vi "DelayFind.vi"() -> ()   [LabVIEW 2020]
doc: "Example Description:\nThis example demonstrates how to enable Time Interleaved Sampling with the NI 5772 adapter module to achieve a sampling rate of 1.6GS/s. This example continuously acquires records of analog input data from the NI 5772 adapter module. It allows you to select an AI channel, trigger type, and record size. This VI must be compiled before it is run. \n\nVI Configuration:\nThis example uses the NI PXI-7952R as the FPGA target by default. If you are using another FPGA target, complete the following steps to configure the host VI to use a VI configured for your FPGA target:\n1. On the block diagram, right-click the Open FPGA VI Reference (NI PXI-7952R) function and select Configure Open FPGA VI Reference.\n2. Browse for a new target by clicking the Browse Project button in the Open VI section.\n3. Select the VI under the target that matches your device. Click OK to select this VI.\n4. Click OK to exit the dialog box and to apply the new selection to the FPGA VI.\n5. Save the VI.\n\nRunning the VI:\n1. Select a RIO Resource that corresponds to the FPGA device configured above.\n2. Clock Configuration: Select the desired clock source for the adapter module.\nAnalog Input: Configure the AI Channel, Record Size, and Trigger Type controls. If you are using the analog trigger type, configure the Trigger Level (V) control.\n3. Click the run arrow to run the VI.\n4. If the Trigger Type is set to Software, click the Software Trigger button to acquire a single record of data. If the Trigger Type is set to Data Edge, a record of data is acquired each time the input signal rises above the trigger level.\n\nThe Record Size, Trigger Type, and Trigger Level (V) controls can all be configured while the VI is running. \n\nNote: The AI Channel control must be configured before the VI is run.\n\nExecution Steps:s\n1. Open a session to the FPGA VI and run the VI.\n2. Wait for the adapter module to load its default configuration.\n3. Configure the NI 5772 for Time Interleaved Sampling (TIS)\n4. The Trigger type and record size for a single record acquisition are configured.\n5. Based on the trigger type, either wait for the software trigger Boolean to assert or configure the desired trigger level and arm the trigger.\n6. After the trigger is armed, a single record of data is acquired and read.\n7. Stop the VI when the stop button is pressed or when an error has occurred. \n8. Close the FPGA VI reference and display any errors."
uses:
  <vilib>/rvi/interface/nirviCloseFPGA/nirviCloseFPGA.xnode
  SubVIs/DigiFPGARef.ctl
  <vilib>/FPGAPlugInAG/Dynamic/niLvFpga_Close_Dynamic.vi
  Gen/Generator_States.ctl
  <instrlib>/_niInstr/Basic Elements/v1/FPGA/niInstr Basic Elements v1 FPGA.lvlib
  Digitizer_StatesMain.ctl
  <vilib>/rvi/interface/nirviReadWriteControl/nirviReadWriteControl.xnode
  <vilib>/rvi/interface/Simulation/niFpgaSimulationCallBeginRW.vi
  <vilib>/rvi/errors/niLvFpgaAdjustHostInterfaceError.vi
  <vilib>/userdefined/High Color/nirio_resource_hc.ctl
panel:
  out "Trigger Count":u32
  out "Digitizer On":bool
  in  "Amplitude Range":cluster{"Slider 1":dbl, "Slider 1":dbl}(slide)={"Slider 1"=1.0, "Slider 1"=1.6299559471365639} scale=-2.5..2.5
  in  "Range":dbl=2.0
  in  "FineDelay  Control":dbl(slide)=1.0 scale=-2.0..2.0
  in  "Amplitude \nAveraging":u16(slide)=1 caption="Amplitude Averaging" scale=0.0..8.0 scale format="%#.2g"
  in  "Time Division":u8(slide)=1 max=2 step=1 scale=0.0..2.0
  out "Gen Actual Sample Rate":dbl format="%#_6p"
  out "TIS Configured?":bool
  out "Configured?":bool
  in  "Record Size":u16=1024
  in  "Delay(us)":sgl min=0 step=0.1 format="%#_4g"
  in  "TrigIn_Sim":bool caption="Pause"
  out "Waveform LIVE":cluster{"Start Time":dbl, dbl, ext[]}(graph)
  in  "Start Digi":bool
  out "Input Waveform 2":waveform(dbl)(graph)
  out "TimeDivFactor":i16
  out "Read Size (Host)":u16
  out "range (Vpp)":dbl=1.3
  out "FPGA VI Reference Out":T1
  in  "Start Gen":bool
  out "Generator On":bool
  out "Input Waveform":dbl[](graph)
  in  "stop Gen":bool
  in  "Stop Generator \nApplication":bool
  out "Waves per Pixel":u32
  out "Sampling Frequency (Hz)":u64
  out "Amplitudes":dbl[](array[numeric]) format="%.2f"
  out "Offset Factor":dbl
  out "Gain":dbl
  in  "Use Default Wave Settings":bool caption="Checkbox"
  in  "Generator Resource":refnum<k15>
  in  "nGenTrig/vi":bool=TRUE caption="Trigger Mode"
  in  "Digi RIO Resource":T2="PXI1Slot2"
  in  "Ext/nViTrig":bool=TRUE
  in  "Send vi Trig":bool
  in  "Trigger Level (V)":dbl
  out "WaveSampleCount":i16=1024
  out "AvgCount_powerOf2":i16(knob) caption="Amplitude Avg" min=0 max=8 step=1 scale=0.0..8.0
  in  "Stop Digi App":bool caption="Stop Digi \nApplication"
  in  "Trigger Type":enum8{"Software", "Data Edge"}(ring)
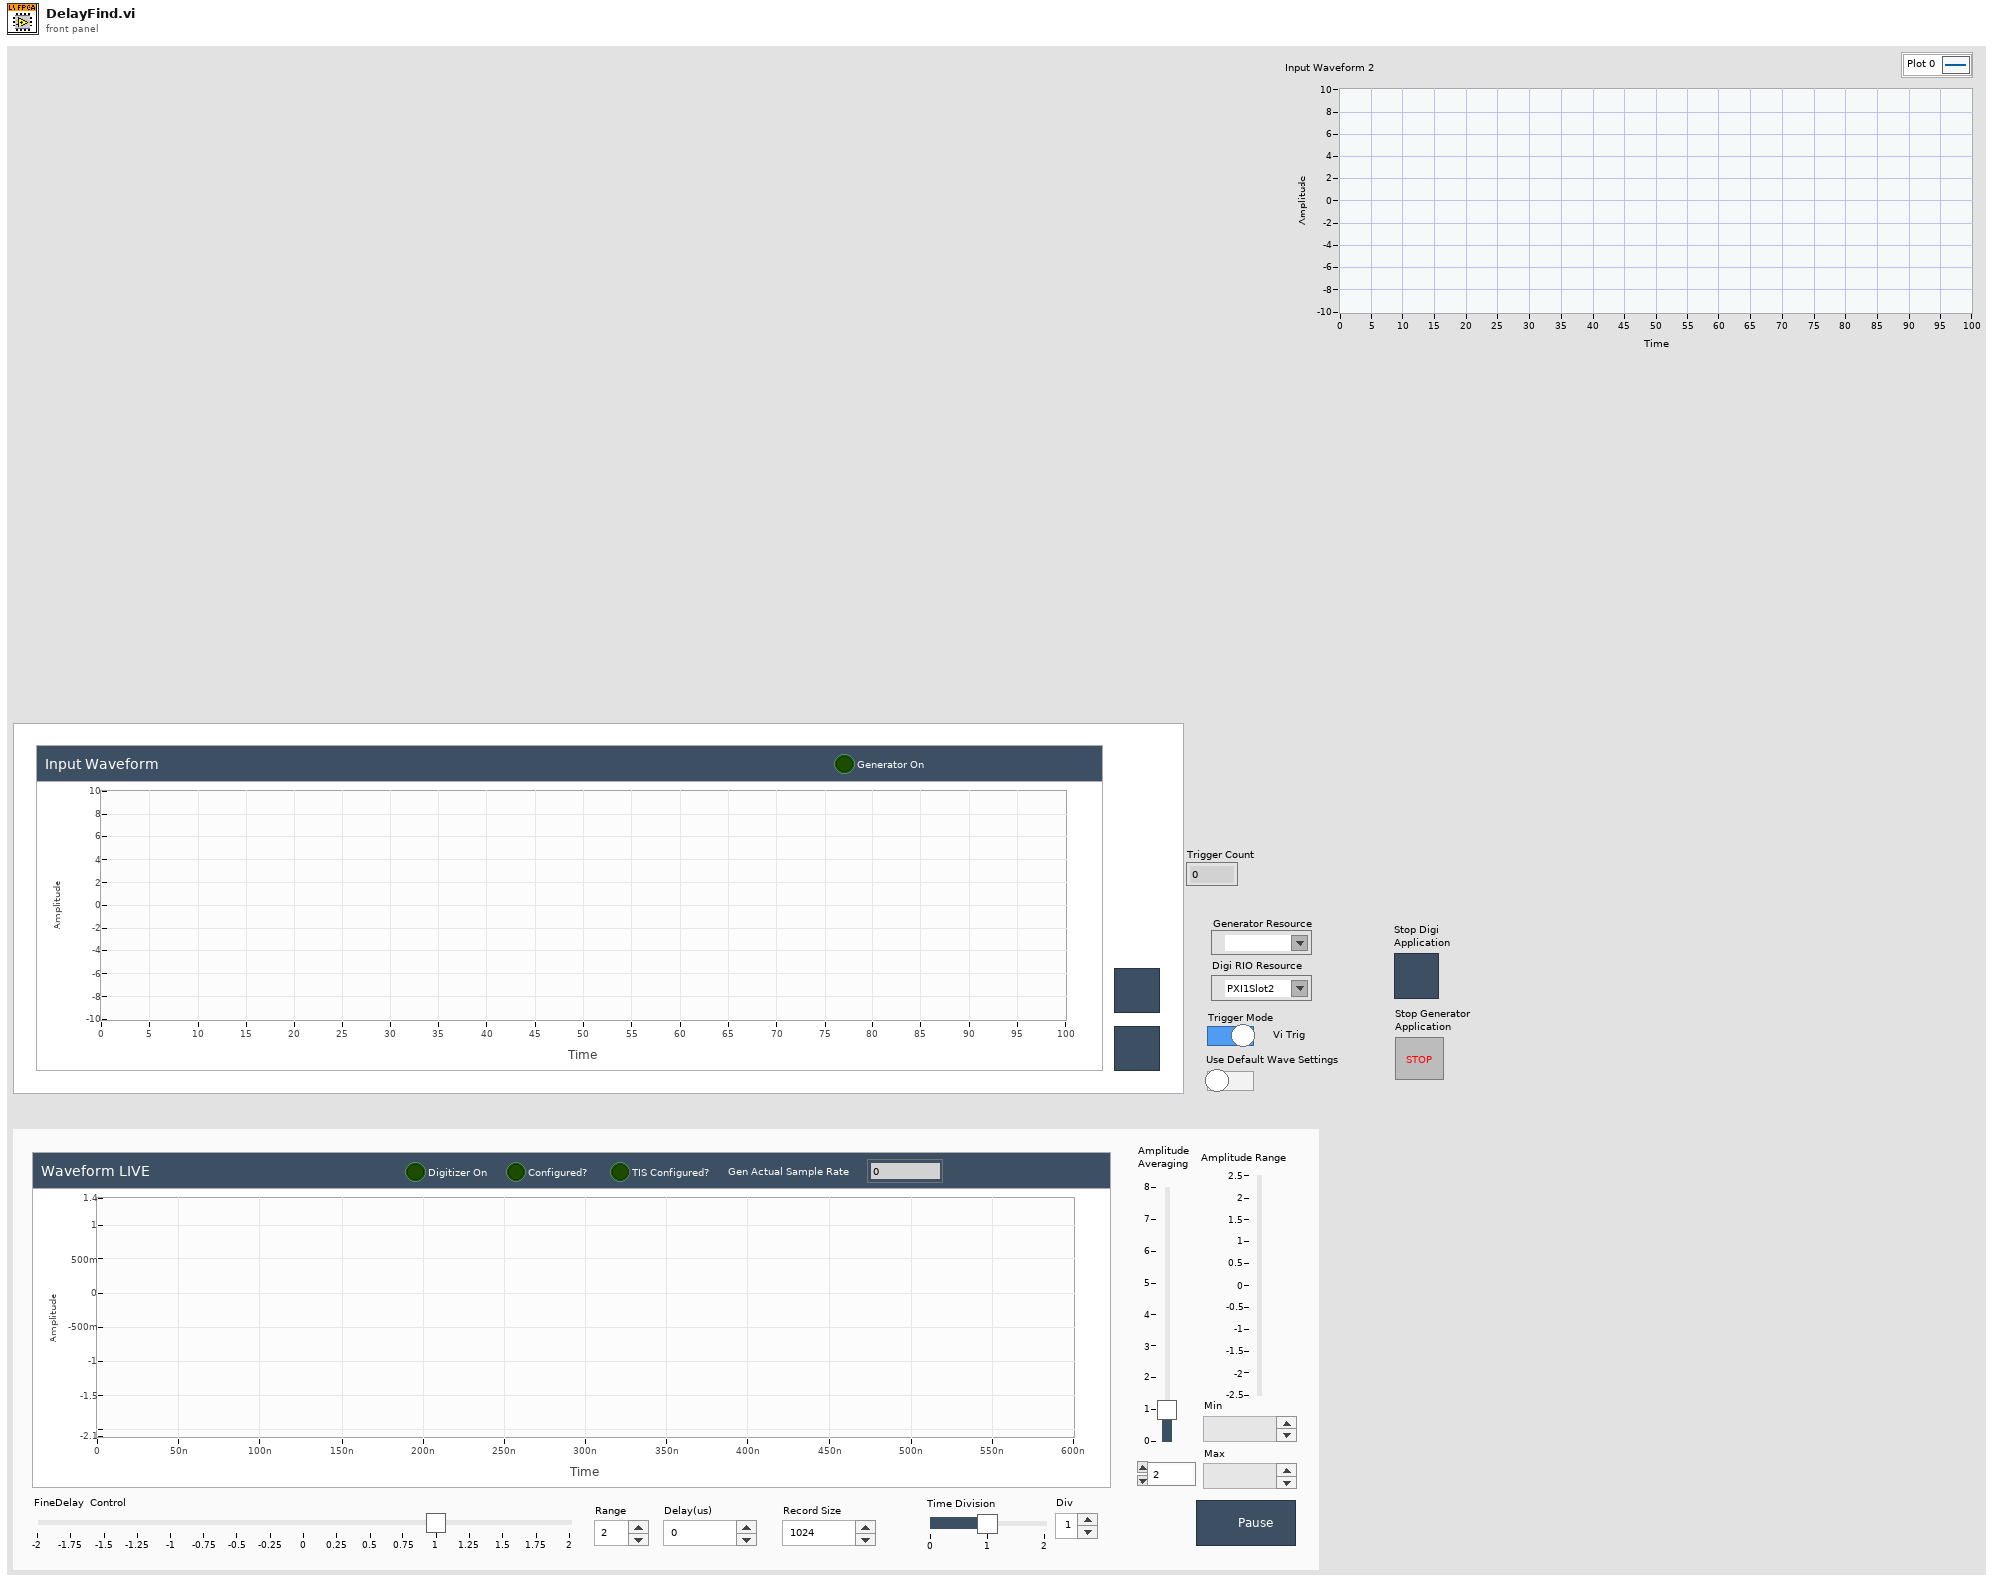
[diagram p1: front panel]
types:
  T1 = typedef "DigiFPGARef.ctl" = refnum<k20>
  T2 = typedef "nirio_resource_hc.ctl" = tag
  T3 = typedef "Digitizer_StatesMain.ctl" = enum16{"Idle", "Init", "SetParam", "Read", "CloseDigi", "CloseApp"}
  T4 = typedef "Generator_States.ctl" = enum16{"Idle", "GenerateWaveArray", "InitGen", "SendVITrig", "CloseGen", "CloseApp"}
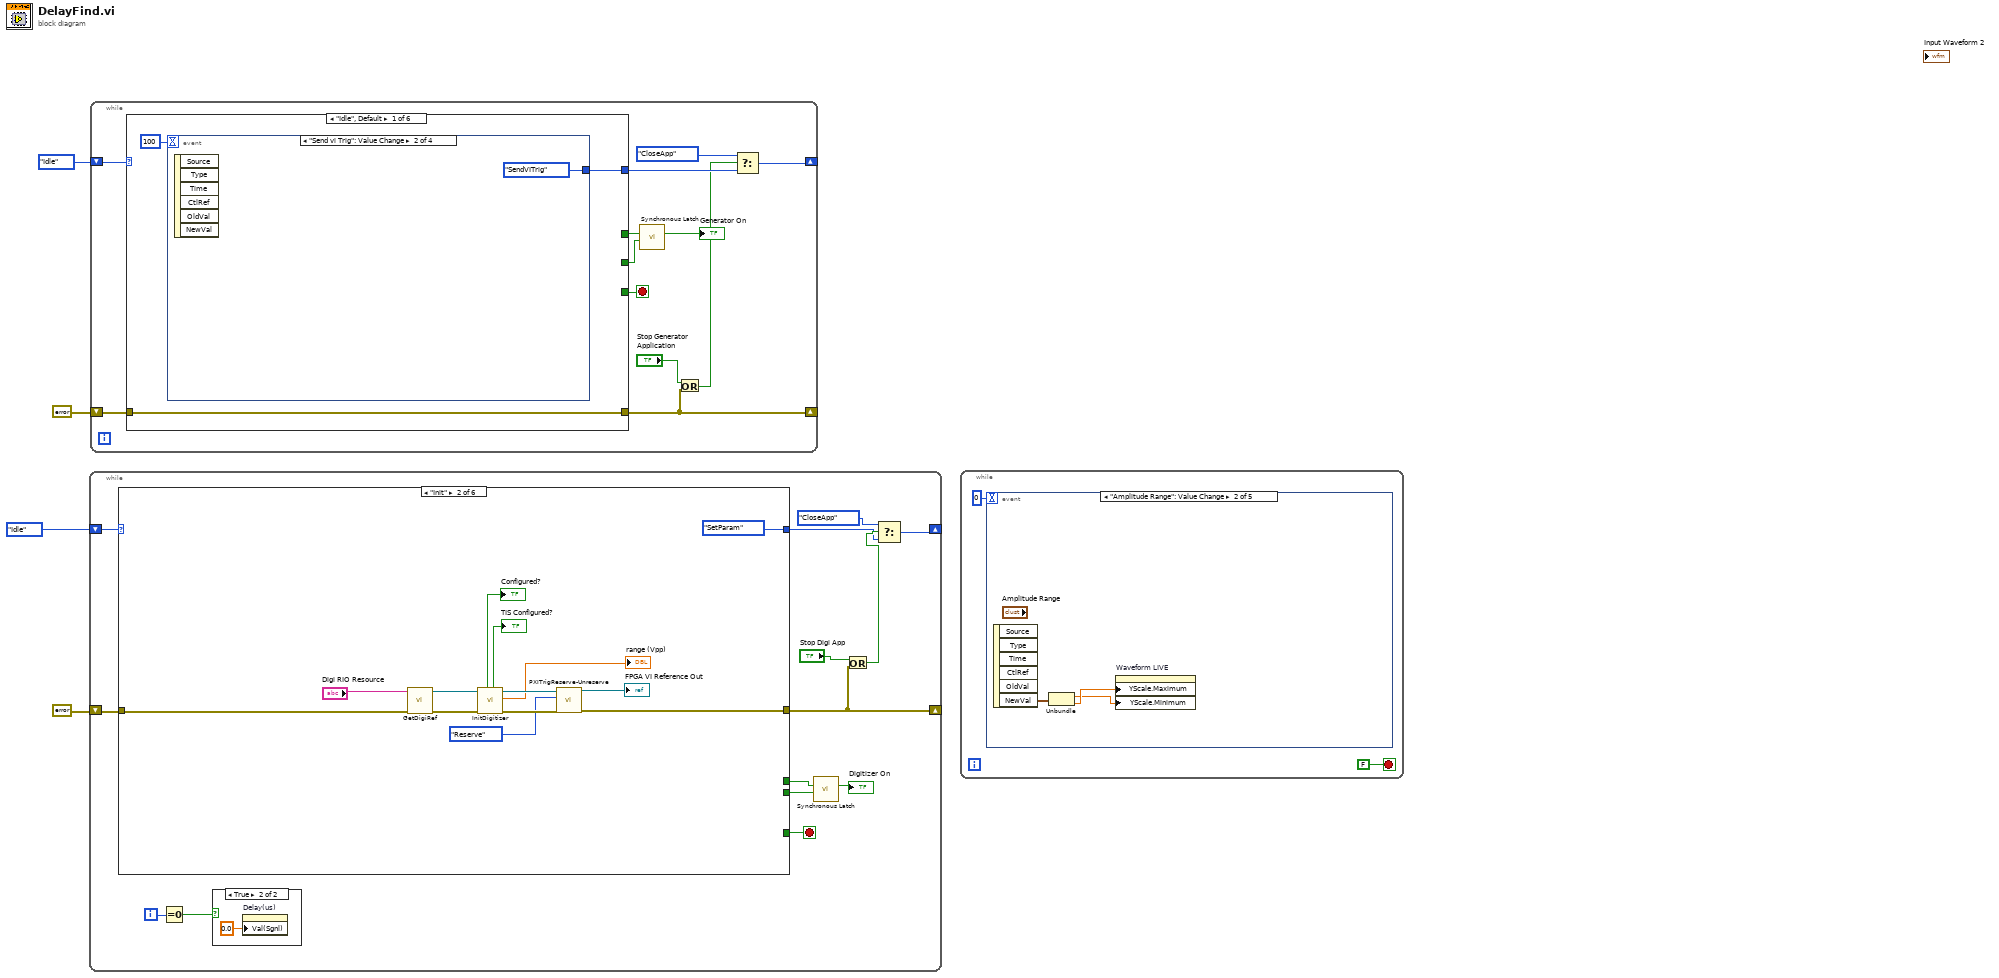
[diagram p0: block diagram]
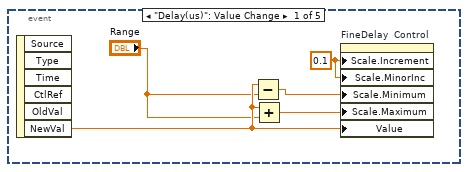
[diagram p2: hidden frame]
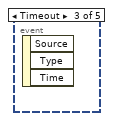
[diagram p3: hidden frame]
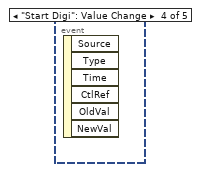
[diagram p4: hidden frame]
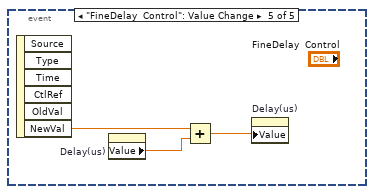
[diagram p5: hidden frame]
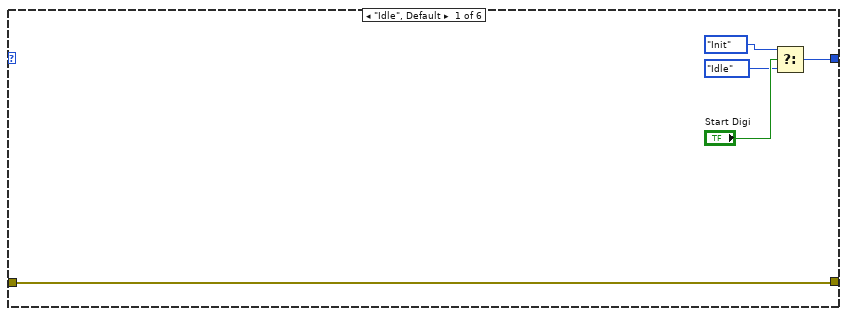
[diagram p7: hidden frame]
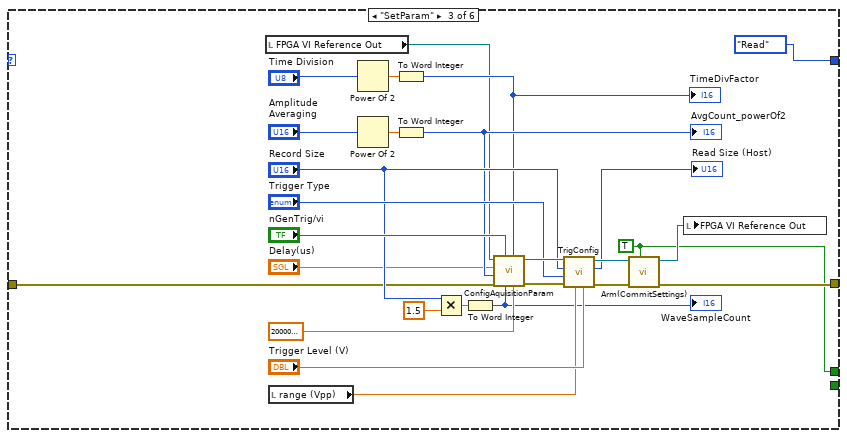
[diagram p8: hidden frame]
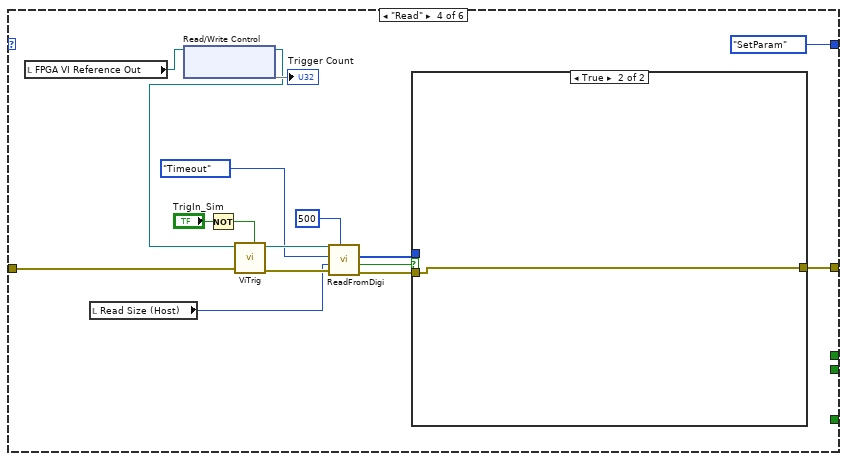
[diagram p9: hidden frame]
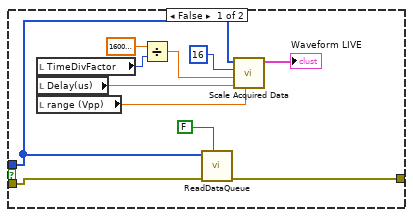
[diagram p10: hidden frame]
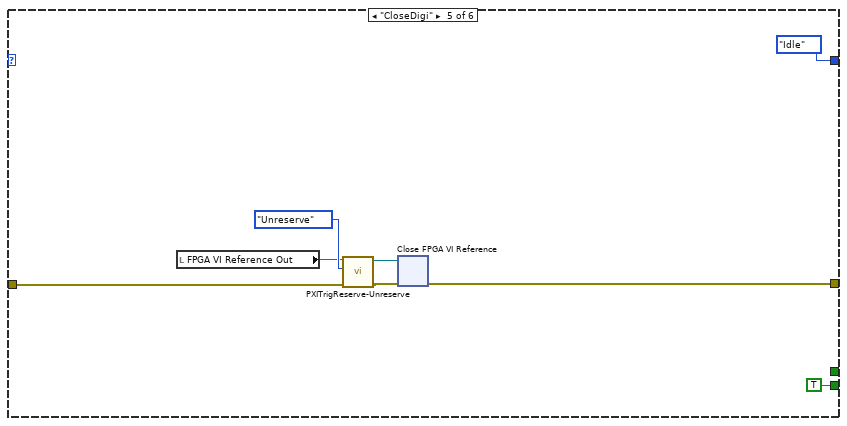
[diagram p11: hidden frame]
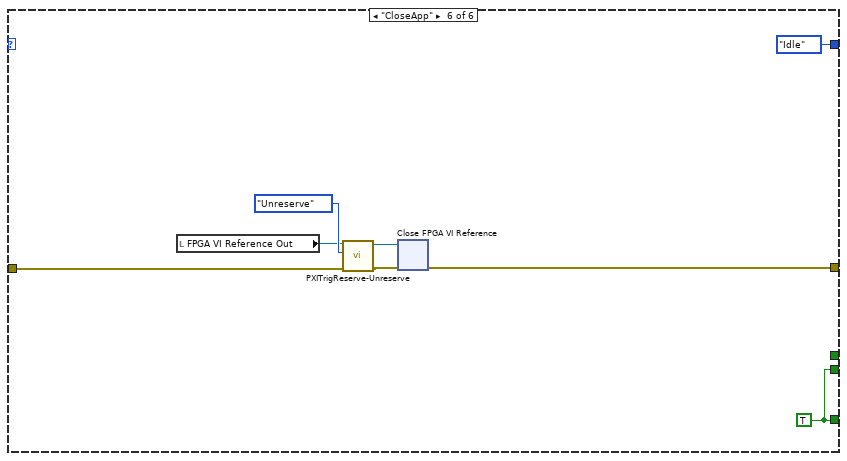
[diagram p12: hidden frame]
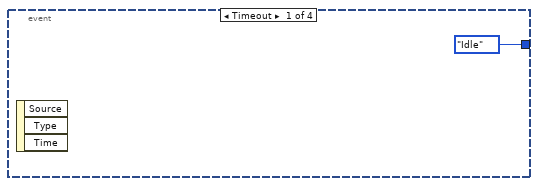
[diagram p13: hidden frame]
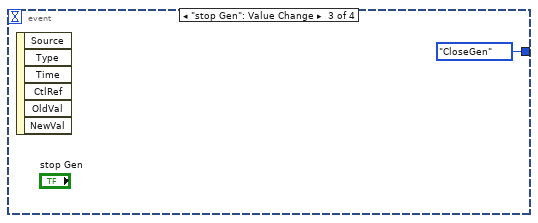
[diagram p14: hidden frame]
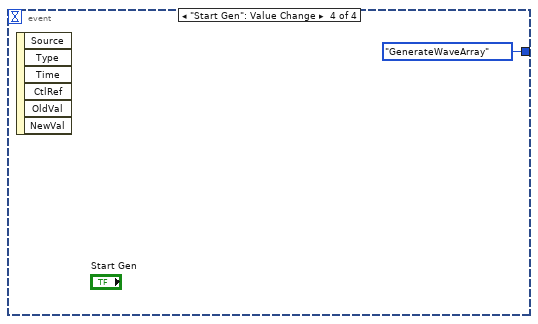
[diagram p15: hidden frame]
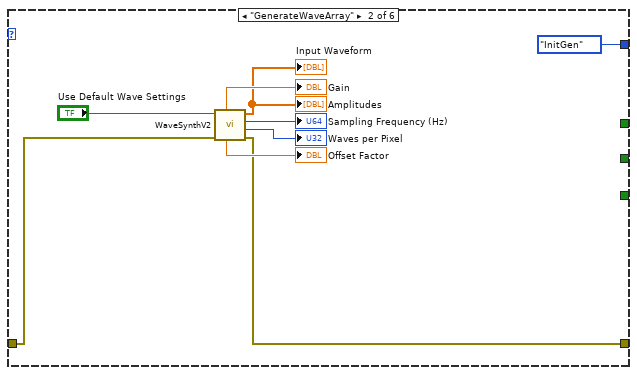
[diagram p16: hidden frame]
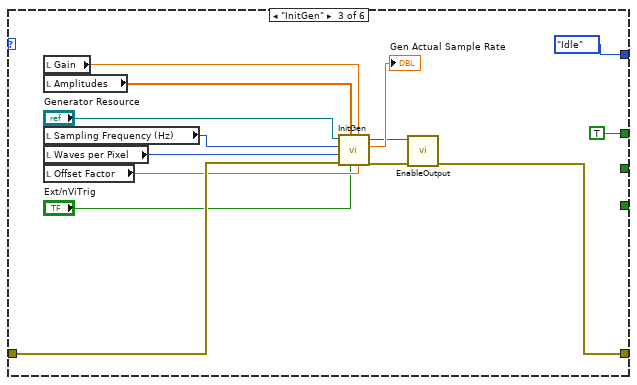
[diagram p17: hidden frame]
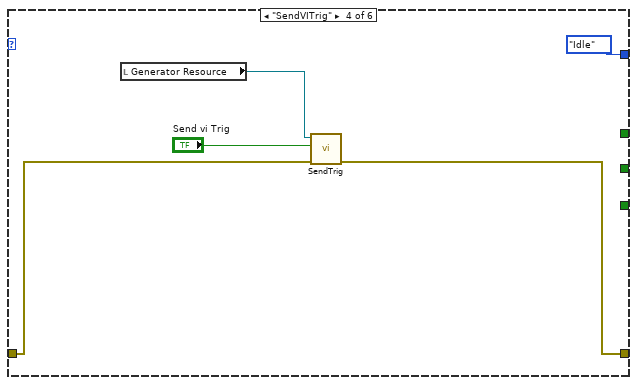
[diagram p18: hidden frame]
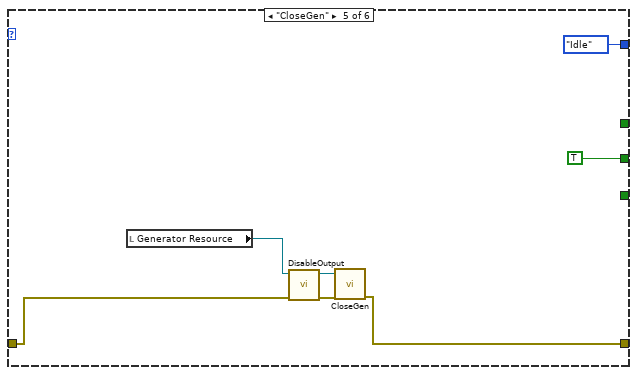
[diagram p19: hidden frame]
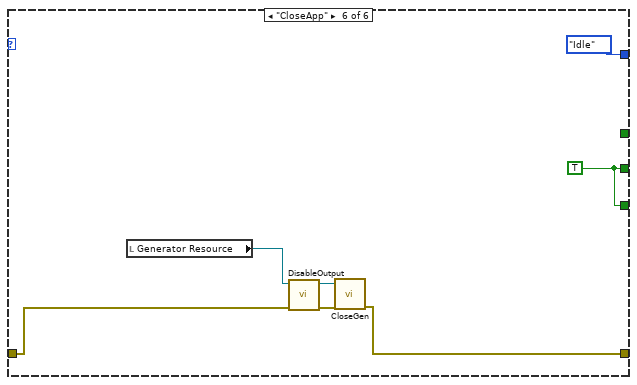
[diagram p20: hidden frame]
diagram:
  n1 = while {
    shift-right: [w13] -> _
    shift-left: Digitizer_StatesMain."Idle" -> [w18]
    shift-right: [w8] -> _
    shift-left: errorcluster {"status"=FALSE, "code"=0, "source"=""} ("error out") -> [w17]
    i -> [w15]
    stop <- w14 stop-if-true
    n2 = case shown="\"Init\"" w18 {
      tunnel: w17 -> [w24 w29 w44 w72 w97 w105]
      tunnel: [w24 w28 w46 w68 w96 w104] -> w8
      tunnel: [w23 Digitizer_StatesMain."SetParam" Digitizer_StatesMain."Read" Digitizer_StatesMain."SetParam" Digitizer_StatesMain."Idle" Digitizer_StatesMain."Idle"] -> w9
      tunnel: [_ _ _ _ _ w101] -> w14
      tunnel: [_ _ _ _ TRUE ("stop") w101] -> w6
      tunnel: [_ _ w38 _ _ _] -> w5
      frame "Idle", Default {
        n3 = Select(t=Digitizer_StatesMain."Init", s="Start Digi", f=Digitizer_StatesMain."Idle") -> (s? t:f=w23:T3)
      }
      frame "Init" {
        n4 = call "GetDigiRef.vi"("error in (no error)"=w29, "RIO Device IN"="Digi RIO Resource") -> ("error out"=w31:errorcluster, "FPGA VI Reference Out"=w36:T1)  [unwired: 8 in]
        n5 = call "InitDigitizer.vi"("error in"=w31, "FPGA VI Reference"=w36) -> ("error out"=w34:errorcluster, "range (Vpp)"=→"range (Vpp)":dbl, "FPGA VI Reference Out"=w33:T1, "TIS Configured?"=→"TIS Configured?":bool, "Configured?"=→"Configured?":bool)  [unwired: 5 in]
        n6 = call "PXITrigReserve-Unreserve.vi"("error in"=w34, "Mode"=enum16{"Reserve", "Unreserve"}."Reserve", "FPGA VI Reference"=w33) -> ("error out"=w28:errorcluster, "FPGA VI Reference Out"=→"FPGA VI Reference Out":T1)  [unwired: 7 in]
      }
      frame "SetParam" {
        w38 = TRUE ("Arm?")
        n7 = local read "FPGA VI Reference Out"() -> (w43:T1)
        n8 = local read "range (Vpp)"() -> (w42:dbl)
        n9 = Power Of 2(x="Time Division") -> (2^x=w58:dbl)
        n10 = Power Of 2(x="Amplitude \nAveraging") -> (2^x=w53:dbl)
        n11 = To Word Integer(number=w58) -> (16bit integer=w48:i16)
        "TimeDivFactor" <- w48
        n12 = To Word Integer(number=w53) -> (16bit integer=w51:i16)
        "AvgCount_powerOf2" <- w51
        n13 = Multiply(x="Record Size", y=sgl 1.5) -> (x*y=w55:sgl)
        n14 = To Word Integer(number=w55) -> (16bit integer=w40:i16)
        "WaveSampleCount" <- w40
        n15 = call "ConfigAquisitionParam.vi"("Wave Sampling Rate"=sgl 200000000.0, "Neighbour Avg"=w48, "WaveSampleCount"=w40, "vi/nGenTrig"="nGenTrig/vi", "error in"=w44, "AvgCount_powerOf2"=w51, "Delay (us)"="Delay(us)", "FPGA VI Reference"=w43) -> ("error out"=w63:errorcluster, "FPGA VI Reference Out"=w64:T1)  [unwired: 2 in]
        n16 = call "TrigConfig.vi"("Trigger Level (V)"="Trigger Level (V)", "range (Vpp)"=w42, "error in"=w63, "Trigger Type"="Trigger Type", "Requested Samples Per Pixel"="Record Size", "FPGA VI Reference"=w64) -> ("error out"=w56:errorcluster, "Read Size (Host)"=→"Read Size (Host)":u16, "FPGA VI Reference Out"=w57:T1)  [unwired: 3 in]
        n17 = call "Arm(CommitSettings).vi"("Arm?"=w38, "error in"=w56, "FPGA VI Reference"=w57) -> ("error out"=w46:errorcluster, "FPGA VI Reference Out"=w39:T1)  [unwired: 7 in]
        n18 = local write "FPGA VI Reference Out"(w39) -> ()
      }
      frame "Read" {
        n19 = local read "FPGA VI Reference Out"() -> (w66:T1)
        n20 = local read "Read Size (Host)"() -> (w70:u16)
        n21 = xnode "Read/Write Control"("FPGA VI Reference In"=w66) -> ("FPGA VI Reference Out"=w65:T1, "Trigger Count"=→"Trigger Count")  [unwired: 1 in, 1 out]
        n22 = Not(x="TrigIn_Sim") -> (.not. x?=w80:bool)
        n23 = call "ViTrig.vi"("Vi Trigger"=w80, "error in"=w72, "FPGA VI Reference"=w65) -> ("error out"=w76:errorcluster, "FPGA VI Reference Out"=w75:T1)  [unwired: 7 in]
        n24 = call "ReadFromDigi.vi"("Timeout (ms)"=500, "error in"=w76, "Number of Elements"=w70, "Mode"=enum16{"Wait For Data", "Timeout"}."Timeout", "FPGA VI Reference"=w75) -> ("error out"=w69:errorcluster, "Error/Timeout?"=w79:bool, "Output Waveform"=w77:u16[])  [unwired: 3 in, 1 out]
        n25 = case shown="True" w79 {
          tunnel: w77 -> [w82 _]
          tunnel: w69 -> [w84 w92]
          tunnel: [w83 w92] -> w68
          frame False {
            n26 = local read "TimeDivFactor"() -> (w85:i16)
            n27 = local read "Delay(us)"() -> (w87:sgl)
            n28 = local read "range (Vpp)"() -> (w86:dbl)
            n29 = Divide(x=1600000000.0 ("Sample Rate"), y=w85) -> (x/y=w89:dbl)
            n30 = call "ReadDataQueue.vi"("Write/nRead"=FALSE, "error in (no error)"=w84, "Output Waveform"=w82) -> ("error out"=w83:errorcluster)  [unwired: 7 in, 1 out]
            n31 = call "Scale Acquired Data.vi"("range (V)"=w86, "Start Time (us)"=w87, "Sample Rate"=w89, "Number of Bits"=i16 16, "Data In"=w82) -> ("output waveform"=→"Waveform LIVE":cluster{"Start Time":dbl, dbl, ext[]})  [unwired: 6 out]
          }
          frame True {
          }
        }
      }
      frame "CloseDigi" {
        n32 = local read "FPGA VI Reference Out"() -> (w95:T1)
        n33 = call "PXITrigReserve-Unreserve.vi"("error in"=w97, "Mode"=enum16{"Reserve", "Unreserve"}."Unreserve", "FPGA VI Reference"=w95) -> ("error out"=w100:errorcluster, "FPGA VI Reference Out"=w99:T1)  [unwired: 7 in]
        n34 = xnode "Close FPGA VI Reference"("FPGA VI Reference In"=w99, "error in"=w100) -> ("error out"=w96:errorcluster)
      }
      frame "CloseApp" {
        w101 = TRUE ("stop")
        n35 = local read "FPGA VI Reference Out"() -> (w103:T1)
        n36 = call "PXITrigReserve-Unreserve.vi"("error in"=w105, "Mode"=enum16{"Reserve", "Unreserve"}."Unreserve", "FPGA VI Reference"=w103) -> ("error out"=w108:errorcluster, "FPGA VI Reference Out"=w107:T1)  [unwired: 7 in]
        n37 = xnode "Close FPGA VI Reference"("FPGA VI Reference In"=w107, "error in"=w108) -> ("error out"=w104:errorcluster)
      }
    }
    n38 = Equal To 0?(x=w15) -> (x = 0?=w16:bool)
    n39 = case shown="True" w16 {
      frame False {
      }
      frame True {
        n40 = property on="Delay(us)" class="DigNum (strict)"("Val(Sgnl)"=sgl 0.0 ("Value (Signaling)")) -> ()  [unwired: 2 in, 2 out]
      }
    }
    n41 = call <instrlib>:"Synchronous Latch.vi"("clear"=w6, "set"=w5) -> ("out"=→"Digitizer On":bool)  [unwired: 9 in]
    n42 = Or(x="Stop Digi App", y=w8) -> (x .or. y?=w10:bool)
    n43 = Select(t=Digitizer_StatesMain."CloseApp", s=w10, f=w9) -> (s? t:f=w13:T3)
  }
  n44 = while {
    shift-right: [w117] -> _
    shift-left: Generator_States."Idle" -> [w120]
    shift-right: [w118] -> _
    shift-left: errorcluster {"status"=FALSE, "code"=0, "source"=""} ("error in") -> [w119]
    stop <- w109 stop-if-true
    n45 = case shown="\"Idle\", Default" w120 {
      tunnel: [w122 Generator_States."InitGen" Generator_States."Idle" Generator_States."Idle" Generator_States."Idle" Generator_States."Idle"] -> w116
      tunnel: w119 -> [w121 w136 w149 w155 w160 w167]
      tunnel: [w121 w130 w140 w154 w159 w166] -> w118
      tunnel: [_ _ TRUE ("Ext/nViTrig") _ _ _] -> w114
      tunnel: [_ _ _ _ TRUE ("x .or. y?") w163] -> w113
      tunnel: [_ _ _ _ _ w163] -> w109
      frame "Idle", Default {
        n46 = event shown="[1] \"Send vi Trig\": Value Change" {
          selector: _ -> [_ _ _ _]
          dyn-events: _ -> [_ _ _ _]
          timeout: 100 -> [_ _ _ _]
          tunnel: [Generator_States."Idle" Generator_States."SendVITrig" Generator_States."CloseGen" Generator_States."GenerateWaveArray"] -> w122
          event Timeout {
            n47 = event-data() -> ()  [unwired: 1 in, 3 out]
          }
          event "Send vi Trig": Value Change {
            n48 = event-data() -> ()  [unwired: 1 in, 6 out]
          }
          event "stop Gen": Value Change {
            n49 = event-data() -> ()  [unwired: 1 in, 6 out]
          }
          event "Start Gen": Value Change {
            n50 = event-data() -> ()  [unwired: 1 in, 6 out]
          }
        }
      }
      frame "GenerateWaveArray" {
        n51 = call "WaveSynthV2.vi"("error in"=w136, "Default Wave"="Use Default Wave Settings") -> ("error out"=w130:errorcluster, "Waves per Pixel"=→"Waves per Pixel":u32, "Sampling Frequency (Hz)"=→"Sampling Frequency (Hz)":u64, "Amplitudes"=→"Amplitudes" →"Input Waveform":dbl[], "Offset Factor"=→"Offset Factor":dbl, "Gain"=→"Gain":dbl)  [unwired: 2 in]
      }
      frame "InitGen" {
        n52 = local read "Gain"() -> (w144:dbl)
        n53 = local read "Amplitudes"() -> (w145:dbl[])
        n54 = local read "Sampling Frequency (Hz)"() -> (w147:u64)
        n55 = local read "Waves per Pixel"() -> (w146:u32)
        n56 = local read "Offset Factor"() -> (w143:dbl)
        n57 = call "InitGen.vi"("Offset"=w143, "Gain"=w144, "Ext/nViTrig"="Ext/nViTrig", "Waveform Data Array"=w145, "error in (no error)"=w149, "Wave Per Pixel"=w146, "Sample Rate (Samp/s)"=w147, "FGEN Resource Name"="Generator Resource") -> ("error out"=w141:errorcluster, "Actual Sample Rate"=→"Gen Actual Sample Rate":dbl, "reference out"=w139:refnum<k15>)  [unwired: 1 in]
        n58 = call "EnableOutput.vi"("error in (no error)"=w141, "FGEN Resource Name"=w139) -> ("error out"=w140:errorcluster)  [unwired: 8 in, 1 out]
      }
      frame "SendVITrig" {
        n59 = local read "Generator Resource"() -> (w151:refnum<k15>)
        n60 = call "SendTrig.vi"("error in (no error)"=w155, "Send vi Trig"="Send vi Trig", "Instrument Handle"=w151) -> ("error out"=w154:errorcluster)  [unwired: 7 in, 1 out]
      }
      frame "CloseGen" {
        n61 = local read "Generator Resource"() -> (w158:refnum<k15>)
        n62 = call "DisableOutput.vi"("error in (no error)"=w160, "FGEN Resource Name"=w158) -> ("error out"=w162:errorcluster, "Instrument Handle Out"=w161:refnum<k15>)  [unwired: 8 in]
        n63 = call "CloseGen.vi"("error in (no error)"=w162, "Instrument Handle"=w161) -> ("error out"=w159:errorcluster)  [unwired: 9 in]
      }
      frame "CloseApp" {
        w163 = TRUE ("x .or. y?")
        n64 = local read "Generator Resource"() -> (w165:refnum<k15>)
        n65 = call "DisableOutput.vi"("error in (no error)"=w167, "FGEN Resource Name"=w165) -> ("error out"=w169:errorcluster, "Instrument Handle Out"=w168:refnum<k15>)  [unwired: 8 in]
        n66 = call "CloseGen.vi"("error in (no error)"=w169, "Instrument Handle"=w168) -> ("error out"=w166:errorcluster)  [unwired: 9 in]
      }
    }
    n67 = call <instrlib>:"Synchronous Latch.vi"("clear"=w113, "set"=w114) -> ("out"=→"Generator On":bool)  [unwired: 9 in]
    n68 = Or(x="Stop Generator \nApplication", y=w118) -> (x .or. y?=w110:bool)
    n69 = Select(t=Generator_States."CloseApp", s=w110, f=w116) -> (s? t:f=w117:T4)
  }
  n70 = while {
    stop <- FALSE stop-if-true
    n71 = event shown="[1] \"Amplitude Range\": Value Change" {
      selector: _ -> [_ _ _ _ _]
      dyn-events: _ -> [_ _ _ _ _]
      timeout: 0 -> [_ _ _ _ _]
      event "Delay(us)": Value Change {
        w176 = 0.1 ("Scale.Range:Increment")
        n72 = event-data() -> ("NewVal"=w173:sgl)  [unwired: 1 in, 5 out]
        n73 = Subtract(x=w173, y="Range") -> (x-y=w175:dbl)
        n74 = Add(x=w173, y="Range") -> (x+y=w174:dbl)
        n75 = property on="FineDelay  Control" class="Slide (strict)"("Scale.Increment"=w176, "Scale.MinorInc"=w176, "Scale.Minimum"=w175, "Scale.Maximum"=w174, "Value"=w173) -> ()  [unwired: 2 in, 2 out]
      }
      event "Amplitude Range": Value Change {
        n76 = event-data() -> ("NewVal"=w179:cluster{"Slider 1":dbl, "Slider 1":dbl})  [unwired: 1 in, 5 out]
        n77 = Unbundle(w179) -> ("Slider 1"=w177:dbl, "Slider 1"=w178:dbl)
        n78 = property on="Waveform LIVE" class="WFGraph (strict)"("YScale.Maximum"=w178, "YScale.Minimum"=w177) -> ()  [unwired: 2 in, 2 out]
      }
      event Timeout {
        n79 = event-data() -> ()  [unwired: 1 in, 3 out]
      }
      event "Start Digi": Value Change {
        n80 = event-data() -> ()  [unwired: 1 in, 6 out]
      }
      event "FineDelay  Control": Value Change {
        n81 = event-data() -> ("NewVal"=w181:dbl)  [unwired: 1 in, 5 out]
        n82 = property on="Delay(us)" class="DigNum (strict)"() -> ("Value"=w182:sgl)  [unwired: 2 in, 2 out]
        n83 = Add(x=w181, y=w182) -> (x+y=w180:dbl)
        n84 = property on="Delay(us)" class="DigNum (strict)"("Value"=w180) -> ()  [unwired: 2 in, 2 out]
      }
    }
  }
